vi "Initialize Shutters.vi"(8 "error in (no error)":errorcluster, 11 "Application in":refnum<class "Application.lvclass">) -> (0 "error out":errorcluster, 3 "Application out":refnum<class "Application.lvclass">)   [LabVIEW 2023, in "Application.lvlib" / "Application.lvclass"]
uses:
  Application.lvclass
  C:/Program Files/National Instruments/LabVIEW 2023/vi.lib/ActorFramework/Actor/Actor.lvclass
  Hardware/NI DAQ/NI DAQ.lvclass
  Application.lvclass/Application.ctl
  User Interface/Splash Screen Messages/Update Status Msg/Update Status Msg.lvclass/Update Status Msg.ctl
  <vilib>/ActorFramework/Message Enqueuer/Message Enqueuer.lvclass/Message Enqueuer.ctl
  <vilib>/ActorFramework/Message Enqueuer/Enqueue.vi
  User Interface/Splash Screen Messages/Update Status Msg/Update Status Msg.lvclass
  C:/Program Files/National Instruments/LabVIEW 2023/vi.lib/ActorFramework/Message/Message.lvclass
  <vilib>/ActorFramework/Message Priority Queue/Priority Enqueue.vi
  <vilib>/ActorFramework/Actor/Actor.lvclass
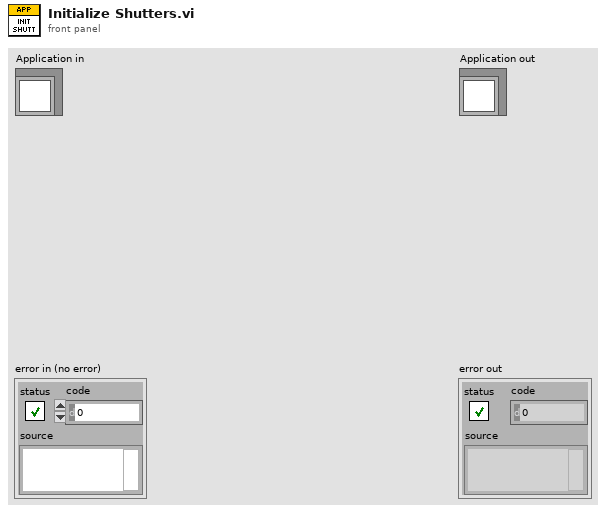
[diagram p1: front panel]
types:
  T1 = typedef "Shutter Configuration.ctl" = cluster{"IO Line":tag, "Name":string, "Wavelength":u16, "Max rate (Hz)":dbl}
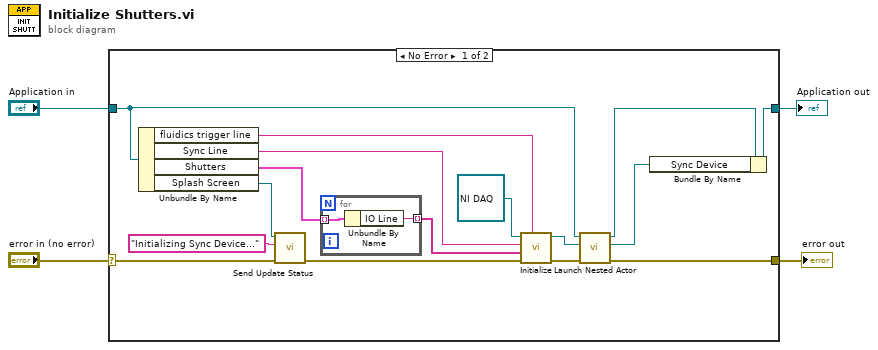
[diagram p0: block diagram]
diagram:
  n1 = case shown="No Error" "error in (no error)" {
    selector: "error in (no error)" -> [w8 w24]
    tunnel: [w18 w24] -> w3
    tunnel: [w19 w23] -> w1
    tunnel: "Application in" -> [w16 w23]
    frame No Error {
      n2 = Unbundle By Name(w16) -> ("fluidics trigger line"=w5:tag, "Sync Line"=w13:tag, "Shutters"=w15:T1[], "Splash Screen"=w6:refnum<class "Message Enqueuer.lvclass">)
      n3 = call "Send Update Status.vi"("error in (no error)"=w8, "Status Message"="Initializing Sync Device...", "Message Enqueuer"=w6) -> ("error out"=w7:errorcluster)  [unwired: 7 in, 1 out]
      n4 = for {
        tunnel: w15 -> [w22] mode=indexing
        tunnel: [w21] -> w14 mode=indexing
        n5 = Unbundle By Name(w22) -> ("IO Line"=w21:tag)
      }
      n6 = call-dynamic "Initialize.vi"("fluidics line"=w5, "error in (no error)"=w7, "Shutter Lines"=w14, "Sync Line"=w13, "Synchronization Device in"=refnum<class "NI DAQ.lvclass"> refnum ("Synchronization Device.lvlib:Synchronization Device.lvclass")) -> ("error out"=w11:errorcluster, "Synchronization Device out"=w12:refnum<class "NI DAQ.lvclass">)  [unwired: 5 in]
      n7 = call <vilib>:"Launch Nested Actor.vi"("error in (no error)"=w11, "Nested Actor"=w12, "Caller Actor in"=w16) -> ("error out"=w18:errorcluster, "Nested Actor's Enqueuer"=w20:refnum<class "Message Enqueuer.lvclass">, "Caller Actor out"=w17:refnum<class "Application.lvclass">)  [unwired: 6 in]
      n8 = Bundle By Name(cluster=w17, "Sync Device"=w20) -> (w19:refnum<class "Application.lvclass">)
    }
    frame Error {
    }
  }
  "error out" <- w3
  "Application out" <- w1
